vi "Write SubVIs.vi"(5 "SubVIs":variant, 9 "PyConvBD in":refnum<class "PyConvBD.lvclass">) -> (3 "PyConvBD out":refnum<class "PyConvBD.lvclass">)   [LabVIEW 2014, in "Raspberry Pi Compatible Compiler for LabVIEW.lvlib" / "PyConvBD.lvclass"]
uses:
  PyConvBD.lvclass
  PyConvBD.lvclass/PyConvBD.ctl
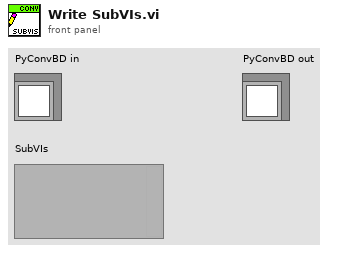
[diagram p1: front panel]
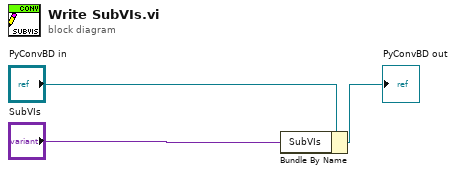
[diagram p0: block diagram]
diagram:
  n1 = Bundle By Name(cluster="PyConvBD in", "SubVIs"="SubVIs") -> (→"PyConvBD out":refnum<class "PyConvBD.lvclass">)
